vi "Do.vi"(8 "error in (no error)":errorcluster, 10 "Actor in":refnum<class "Actor.lvclass">, 11 "Instrument Msg":refnum<class "Instrument Msg.lvclass">) -> (0 "error out":errorcluster, 2 "Actor out":refnum<class "Actor.lvclass">)   [LabVIEW 2020, in "Instrument Handler.lvlib" / "Instrument Msg.lvclass"]
doc: "This implementation will send itself the to the Instrument Handler from where it will be further forwarded."
uses:
  Instrument Msg.lvclass
  C:/Current projects/WS/PPL/HDH.Actor Framework.Core.Publisher.lvlibp/Messages/Response Msg/Response Msg.lvclass
  PPL/HDH.Actor Framework.Core.Actor.lvlibp/1abvi3w/vi.lib/ActorFramework/Actor/Actor.lvclass
  Instrument Owner/Instrument Owner.lvclass
  Multi Instrument Handler/Multi Instrument Handler.lvclass
  Instrument Handler/Instrument Handler.lvclass
  Instrument Msg.lvclass/Instrument Msg.ctl
  PPL/HDH.Actor Framework.Core.Publisher.lvlibp/Publisher Messages/Targetted Msg/Targetted Msg.lvclass
  C:/Current projects/WS/PPL/HDH.Actor Framework.Core.Publisher.lvlibp/Publisher Messages/Sender Msg/Sender Msg.lvclass
  PPL/HDH.Actor Framework.Core.Publisher.lvlibp/Messages/Timed Msg/Timed Msg.lvclass
  PPL/HDH.Actor Framework.Core.Publisher.lvlibp/Messages/Response Msg/Response Msg.lvclass
  C:/Current projects/WS/PPL/HDH.Actor Framework.Core.Actor.lvlibp/1abvi3w/vi.lib/ActorFramework/Actor/Actor.lvclass
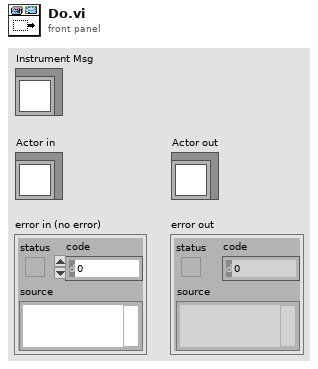
[diagram p1: front panel]
types:
  T1 = typedef "HDH.Actor Framework.Core.Publisher.lvlibp/Ctl_SendFunction.ctl" = enum16{"Send and Forget", "Request Reply", "Await Reply"}
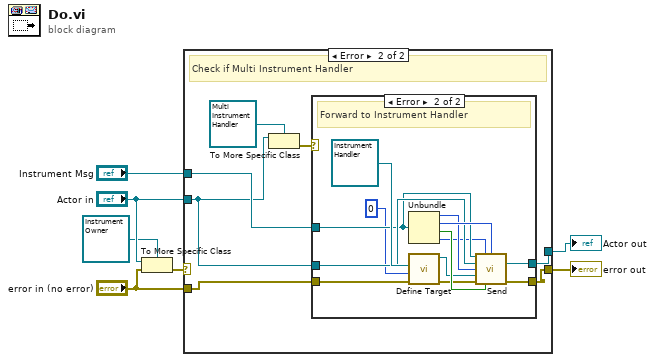
[diagram p0: block diagram]
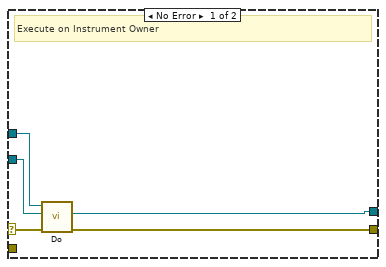
[diagram p2: hidden frame]
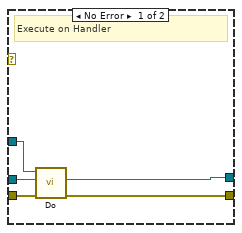
[diagram p3: hidden frame]
diagram:
  n1 = To More Specific Class(target class=refnum<class "Instrument Owner.lvclass"> refnum ("Instrument Handler.lvlib:Instrument Owner.lvclass"), reference="Actor in", error in="error in (no error)") -> (error out=w4:errorcluster)  [unwired: 1 out]
  n2 = case shown="Error" w4 {
    selector: w4 -> [w9 _]
    tunnel: [w12 w17] -> w7
    tunnel: [w11 w18] -> w6
    tunnel: "Instrument Msg" -> [w10 w16]
    tunnel: "Actor in" -> [w8 w15]
    tunnel: "error in (no error)" -> [_ w19]
    frame No Error {
      # "Execute on Instrument Owner"
      n3 = call-parent "Do.vi"("error in (no error)"=w9, "Actor in"=w8, "Response Msg"=w10) -> ("error out"=w12:errorcluster, "Actor out"=w11:refnum<class "Actor.lvclass">)  [unwired: 7 in]
    }
    frame Error {
      # "Check if Multi Instrument Handler"
      n4 = To More Specific Class(target class=refnum<class "Multi Instrument Handler.lvclass"> refnum ("Instrument Handler.lvlib:Multi Instrument Handler.lvclass"), reference=w15) -> (error out=w13:errorcluster)  [unwired: 1 in, 1 out]
      n5 = case shown="Error" w13 {
        tunnel: w19 -> [w21 w34]
        tunnel: w15 -> [w24 w31]
        tunnel: [w22 w29] -> w18
        tunnel: [w20 w28] -> w17
        tunnel: w16 -> [w23 w27]
        frame No Error {
          # "Execute on Handler"
          n6 = call-parent "Do.vi"("error in (no error)"=w21, "Actor in"=w24, "Response Msg"=w23) -> ("error out"=w20:errorcluster, "Actor out"=w22:refnum<class "Actor.lvclass">)  [unwired: 7 in]
        }
        frame Error {
          # "Forward to Instrument Handler"
          n7 = Unbundle(w27) -> (w32:T1, w37:i32, w36:bool, w25:u16)
          n8 = call "Define Target.vi"("error in (no error)"=w34, "Target Actor index(-1, all)"=0, "Target Actor"=refnum<class "Instrument Handler.lvclass"> refnum ("Instrument Handler.lvlib:Instrument Handler.lvclass")) -> ("error out"=w30:errorcluster, "Targetted Msg out"=w33:refnum<class "Targetted Msg.lvclass">)  [unwired: 7 in]
          n9 = call "Send.vi"("Response Msg in"=w27, "Message Priority (Normal)"=w25, "Timeout if waiting(-1ms)"=w37, "Actor in"=w31, "Send Function"=w32, "Sender (publish)"=w33, "error in (no error)"=w30, "Publish Data?(F)"=w36) -> ("Actor out"=w29:refnum<class "Actor.lvclass">, "error out"=w28:errorcluster)  [unwired: 3 in, 3 out]
        }
      }
    }
  }
  "error out" <- w7
  "Actor out" <- w6
